vi "SetRAMFlowRateSetpoint.vi"(7 "Timeout (ms)":u32=2000, 8 "Error In":errorcluster, 10 "Setpoint (mL/min)":dbl format="%.1f", 11 "Sierra M100 In":refnum<visa-resource-name>) -> (0 "Error Out":errorcluster, 2 "Set?":bool, 3 "Sierra M100 Out":refnum<visa-resource-name>)   [LabVIEW 2012, in "Sierra-M100.lvlib"]
doc: "This VI sets the flow rate setpoint in random access memory (RAM). RAM is volatile and this setpoint will NOT be retained after power cycling. Use \"Set Flash Flow Rate Setpoint\" VI instead."
uses:
  Sierra-M100.lvlib
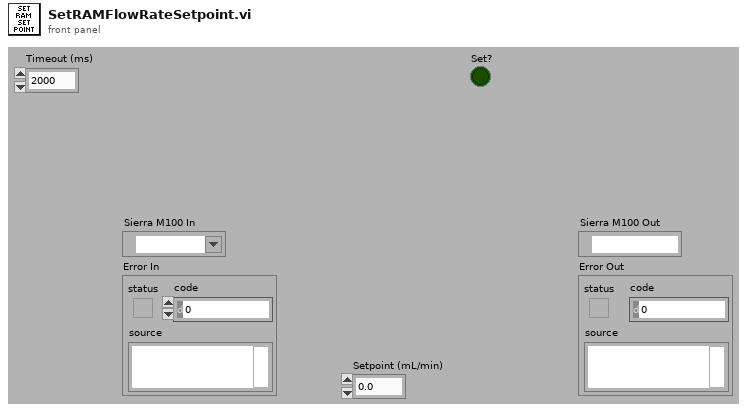
[diagram p1: front panel]
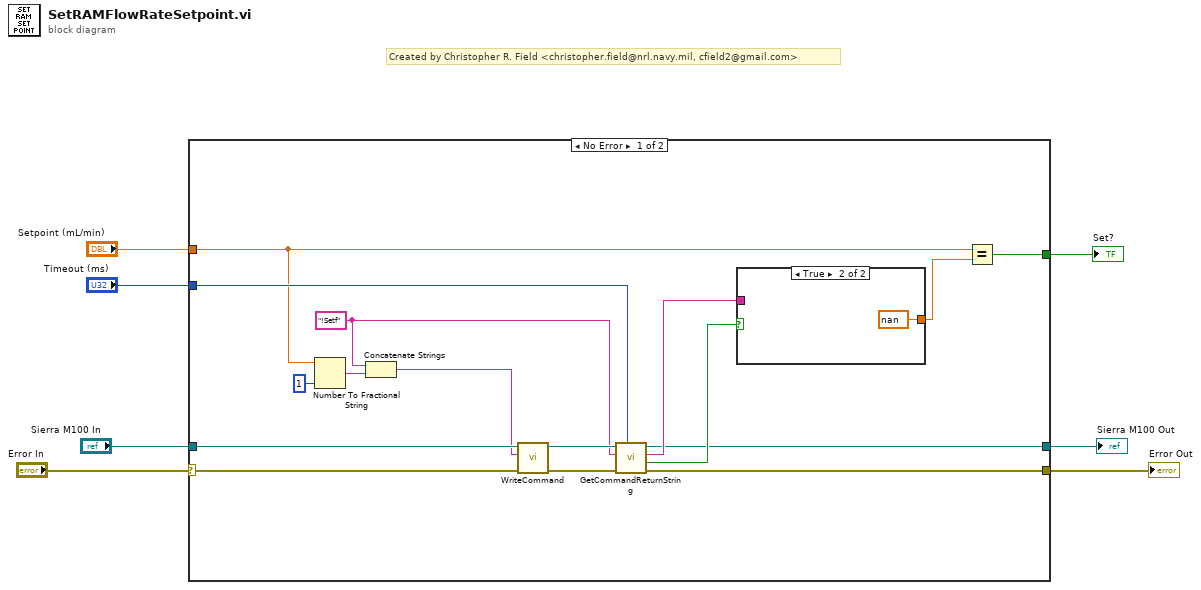
[diagram p0: block diagram]
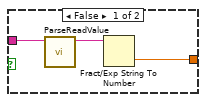
[diagram p2: hidden frame]
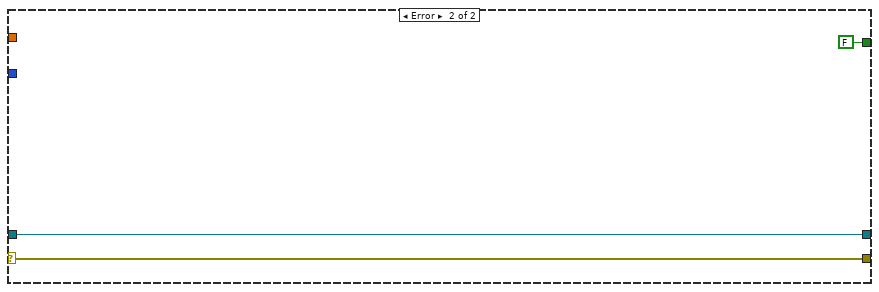
[diagram p3: hidden frame]
diagram:
  # "Created by Christopher R. Field <christopher.field@nrl.navy.mil, cfield2@gmail.com>"
  n1 = case shown="No Error" "Error In" {
    selector: "Error In" -> [w8 w29]
    tunnel: "Sierra M100 In" -> [w21 w30]
    tunnel: "Timeout (ms)" -> [w16 _]
    tunnel: "Setpoint (mL/min)" -> [w12 _]
    tunnel: [w11 FALSE] -> w4
    tunnel: [w10 w30] -> w3
    tunnel: [w9 w29] -> w2
    frame No Error {
      w17 = "!Setf"
      n2 = Number To Fractional String(number=w12, precision (6)=i16 1) -> (F-format string=w22:string)  [unwired: 2 in]
      n3 = Concatenate Strings(w17, w22) -> (w20:string)
      n4 = call "WriteCommand.vi"("Error In"=w8, "Command"=w20, "Smart Trak 2 In"=w21) -> ("Error Out"=w18:errorcluster, "Smart Trak 2 Out"=w19:refnum<visa-resource-name>)  [unwired: 5 in, 2 out]
      n5 = call "GetCommandReturnString.vi"("Timeout (ms)"=w16, "Error In"=w18, "Command"=w17, "Smart Trak 2 In"=w19) -> ("Error Out"=w9:errorcluster, "Timeout?"=w15:bool, "Return String"=w14:string, "Smart Trak 2 Out"=w10:refnum<visa-resource-name>)  [unwired: 4 in]
      n6 = case shown="True" w15 {
        tunnel: w14 -> [w26 _]
        tunnel: [w24 nan] -> w13
        frame False {
          n7 = call "ParseReadValue.vi"("Read Buffer"=w26) -> ("Value"=w25:string)  [unwired: 10 in]
          n8 = Fract/Exp String To Number(string=w25) -> (number=w24:dbl)  [unwired: 3 in, 1 out]
        }
        frame True {
        }
      }
      n9 = Equal?(x=w12, y=w13) -> (x = y?=w11:bool)
    }
    frame Error {
    }
  }
  "Sierra M100 Out" <- w3
  "Error Out" <- w2
  "Set?" <- w4
